vi "Teleop.vi"(8 "Ramps":bool, 9 "Shift":bool, 10 "Match Info":T1={"Autonomous Elapsed Seconds"=0.0, "TeleOp Elapsed Seconds"=0.0, "Disabled Elapsed Seconds"=0.0, "Visited Autonomous"=FALSE, "Visited TeleOp"=FALSE, "Visited Disabled"=FALSE, "Autonomous Settings"={"Autonomous Style"=enum."Independent", "VI Refnum"=refnum}}, 11 "Call Context":T2) -> ()   [LabVIEW 2017]
doc: "This VI is called for each TeleOp packet received from the DS where the robot is not disabled. It is often used to read from the joysticks and update I/O or to update setpoints for timed control loops. It should complete and return within 20 milliseconds or it may miss DS packets."
uses:
  <vilib>/Rock Robotics/WPI/DriverStation/WPI_DriverStationDerivedRobotMode.ctl
  <vilib>/Rock Robotics/WPI/DriverStation/WPI_DriverStationMatch Info.ctl
  <vilib>/Rock Robotics/WPI/Solenoid/WPI_SolenoidValue.ctl
  Public/Documents/Cross The Road Electronics/Phoenix-LabVIEW/Motor Controller/Controls/CTRE_Phoenix_MotorControl_ControlMode.ctl
  <vilib>/Rock Robotics/WPI/Utilities/WPI_GetSetVariantRefNum.vi
  <vilib>/Rock Robotics/Network Tables/NT Write Boolean Array.vi
  <vilib>/Rock Robotics/Network Tables/NT Write Numeric Array.vi
  <vilib>/Rock Robotics/Network Tables/NT Read Boolean.vi
  <vilib>/Rock Robotics/Network Tables/NT Read Numeric Array.vi
  <vilib>/Rock Robotics/Network Tables/NT Read Boolean Array.vi
  <vilib>/Rock Robotics/Network Tables/NT Write Number.vi
  <vilib>/Rock Robotics/WPI/Joystick/WPI_JoystickArcadeMapping.vi
  <vilib>/Rock Robotics/WPI/RobotDrive/WPI_RobotDriveArcadeDrive_Standard(NoSaturation).vi
  <vilib>/Rock Robotics/WPI/ThirdParty/Phoenix-LabVIEW/Motor Controller/Controls/CTRE_Phoenix_MotorControl_NeutralMode.ctl
panel:
  out "element":dbl
  in  "L Retract Ramps":bool
  in  "R Retract Ramps":bool
  in  "RRamp Raise":bool
  in  "LRamp Raise":bool=TRUE
  in  "RRamp Deploy":bool
  in  "LRamp Deploy":bool
  in  "Cube Down":bool
  in  "Cube Up":bool
  in  "Direction Toggle":bool
  in  "Gear Shift":bool
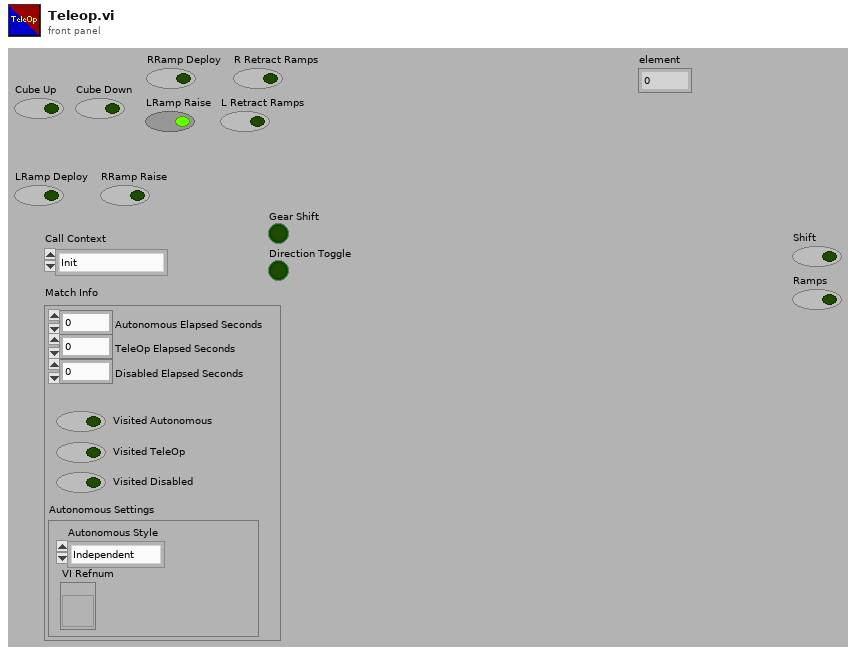
[diagram p1: front panel]
types:
  T1 = typedef "WPI_DriverStationMatch Info.ctl" = cluster{"Autonomous Elapsed Seconds":dbl, "TeleOp Elapsed Seconds":dbl, "Disabled Elapsed Seconds":dbl, "Visited Autonomous":bool, "Visited TeleOp":bool, "Visited Disabled":bool, "Autonomous Settings":cluster{"Autonomous Style":enum16{"Iterative", "Independent"}, "VI Refnum":refnum<vi>}}
  T2 = typedef "WPI_DriverStationDerivedRobotMode.ctl" = enum16{"Init", "Execute", "Stop"}
  T3 = typedef "CTRE_Phoenix_MotorControl_ControlMode.ctl" = u16
  T4 = typedef "WPI_SolenoidValue.ctl" = enum16{"Off", "On", "Forward", "Reverse"}
  T5 = typedef "WPI_JoystickDevRef.ctl" = cluster{"Device":T6}
  T6 = typedef "WPI_JoystickDeviceEnum.ctl" = enum16{"USB 0", "USB 1", "USB 2", "USB 3", "USB 4", "USB 5"}
  T7 = typedef "CTRE_Phoenix_MotorControl_NeutralMode.ctl" = enum8{"EEPROMSetting", "Override to Coast", "Override to Brake"}
  T8 = typedef "WPI_MotorControlDeviceRef.ctl" = cluster{"DeviceStatus":errorcluster, "Type":T9, "PWM":cluster{"PWM Channel":T10, "DeadBand":T11}, "CAN":cluster{"Device Number":u8, "SetOutput VI Ref":variant, "GetOutput VI Ref":variant, "Enable VI Ref":variant, "Disable VI Ref":variant, "Data":variant}, "Invert":bool, "DIO PWM":cluster{"PWM \"Enable\" Channel":T10, "DIOChannel":T12, "PWM Rate":dbl}}
  T9 = typedef "WPI_MotorControlType.ctl" = enum16{"PWM", "CAN", "DIO PWM"}
  T10 = typedef "FPGA_DIOPWMChannel.ctl" = enum8{"PWM 0", "PWM 1", "PWM 2", "PWM 3", "PWM 4", "PWM 5", "PWM 6", "PWM 7", "PWM 8", "PWM 9", "PWM MXP 0", "PWM MXP 1", "PWM MXP 2", "PWM MXP 3", "PWM MXP 4", "PWM MXP 5", "PWM MXP 6", "PWM MXP 7", "PWM MXP 8", "PWM MXP 9", "Invalid"}
  T11 = typedef "WPI_PWMDeadband.ctl" = cluster{"Name":string, "maxPositivePwm":i32, "minPositivePwm":i32, "centerPwm":i32, "maxNegativePwm":i32, "minNegativePwm":i32, "angularRange":u16}
  T12 = typedef "FPGA_DIOChannel.ctl" = enum8{"DIO 0", "DIO 1", "DIO 2", "DIO 3", "DIO 4", "DIO 5", "DIO 6", "DIO 7", "DIO 8", "DIO 9", "DIO MXP 0", "DIO MXP 1", "DIO MXP 2", "DIO MXP 3", "DIO MXP 4", "DIO MXP 5", "DIO MXP 6", "DIO MXP 7", "DIO MXP 8", "DIO MXP 9", "DIO MXP 10", "DIO MXP 11", "DIO MXP 12", "DIO MXP 13", "DIO MXP 14", "DIO MXP 15", "SPI Port CS1", "SPI Port CS2", "SPI Port CS3", "SPI Port MISO", "SPI Port MOSI", "Invalid"}
  T13 = typedef "WPI_RobotDriveDevRef.ctl" = cluster{"DevStatus":errorcluster, "Motors[]":T8[], "Square Inputs":bool, "Max Output":dbl}
  T14 = typedef "WPI_SolenoidDevRef.ctl" = cluster{"DevStatus":errorcluster, "Pneumatics Control Module":u8, "Forward Solenoid Channel":T15, "Reverse Solenoid Channel":T15}
  T15 = typedef "WPI_SolenoidChannel.ctl" = enum8{"Solenoid 0", "Solenoid 1", "Solenoid 2", "Solenoid 3", "Solenoid 4", "Solenoid 5", "Solenoid 6", "Solenoid 7", "Invalid"}
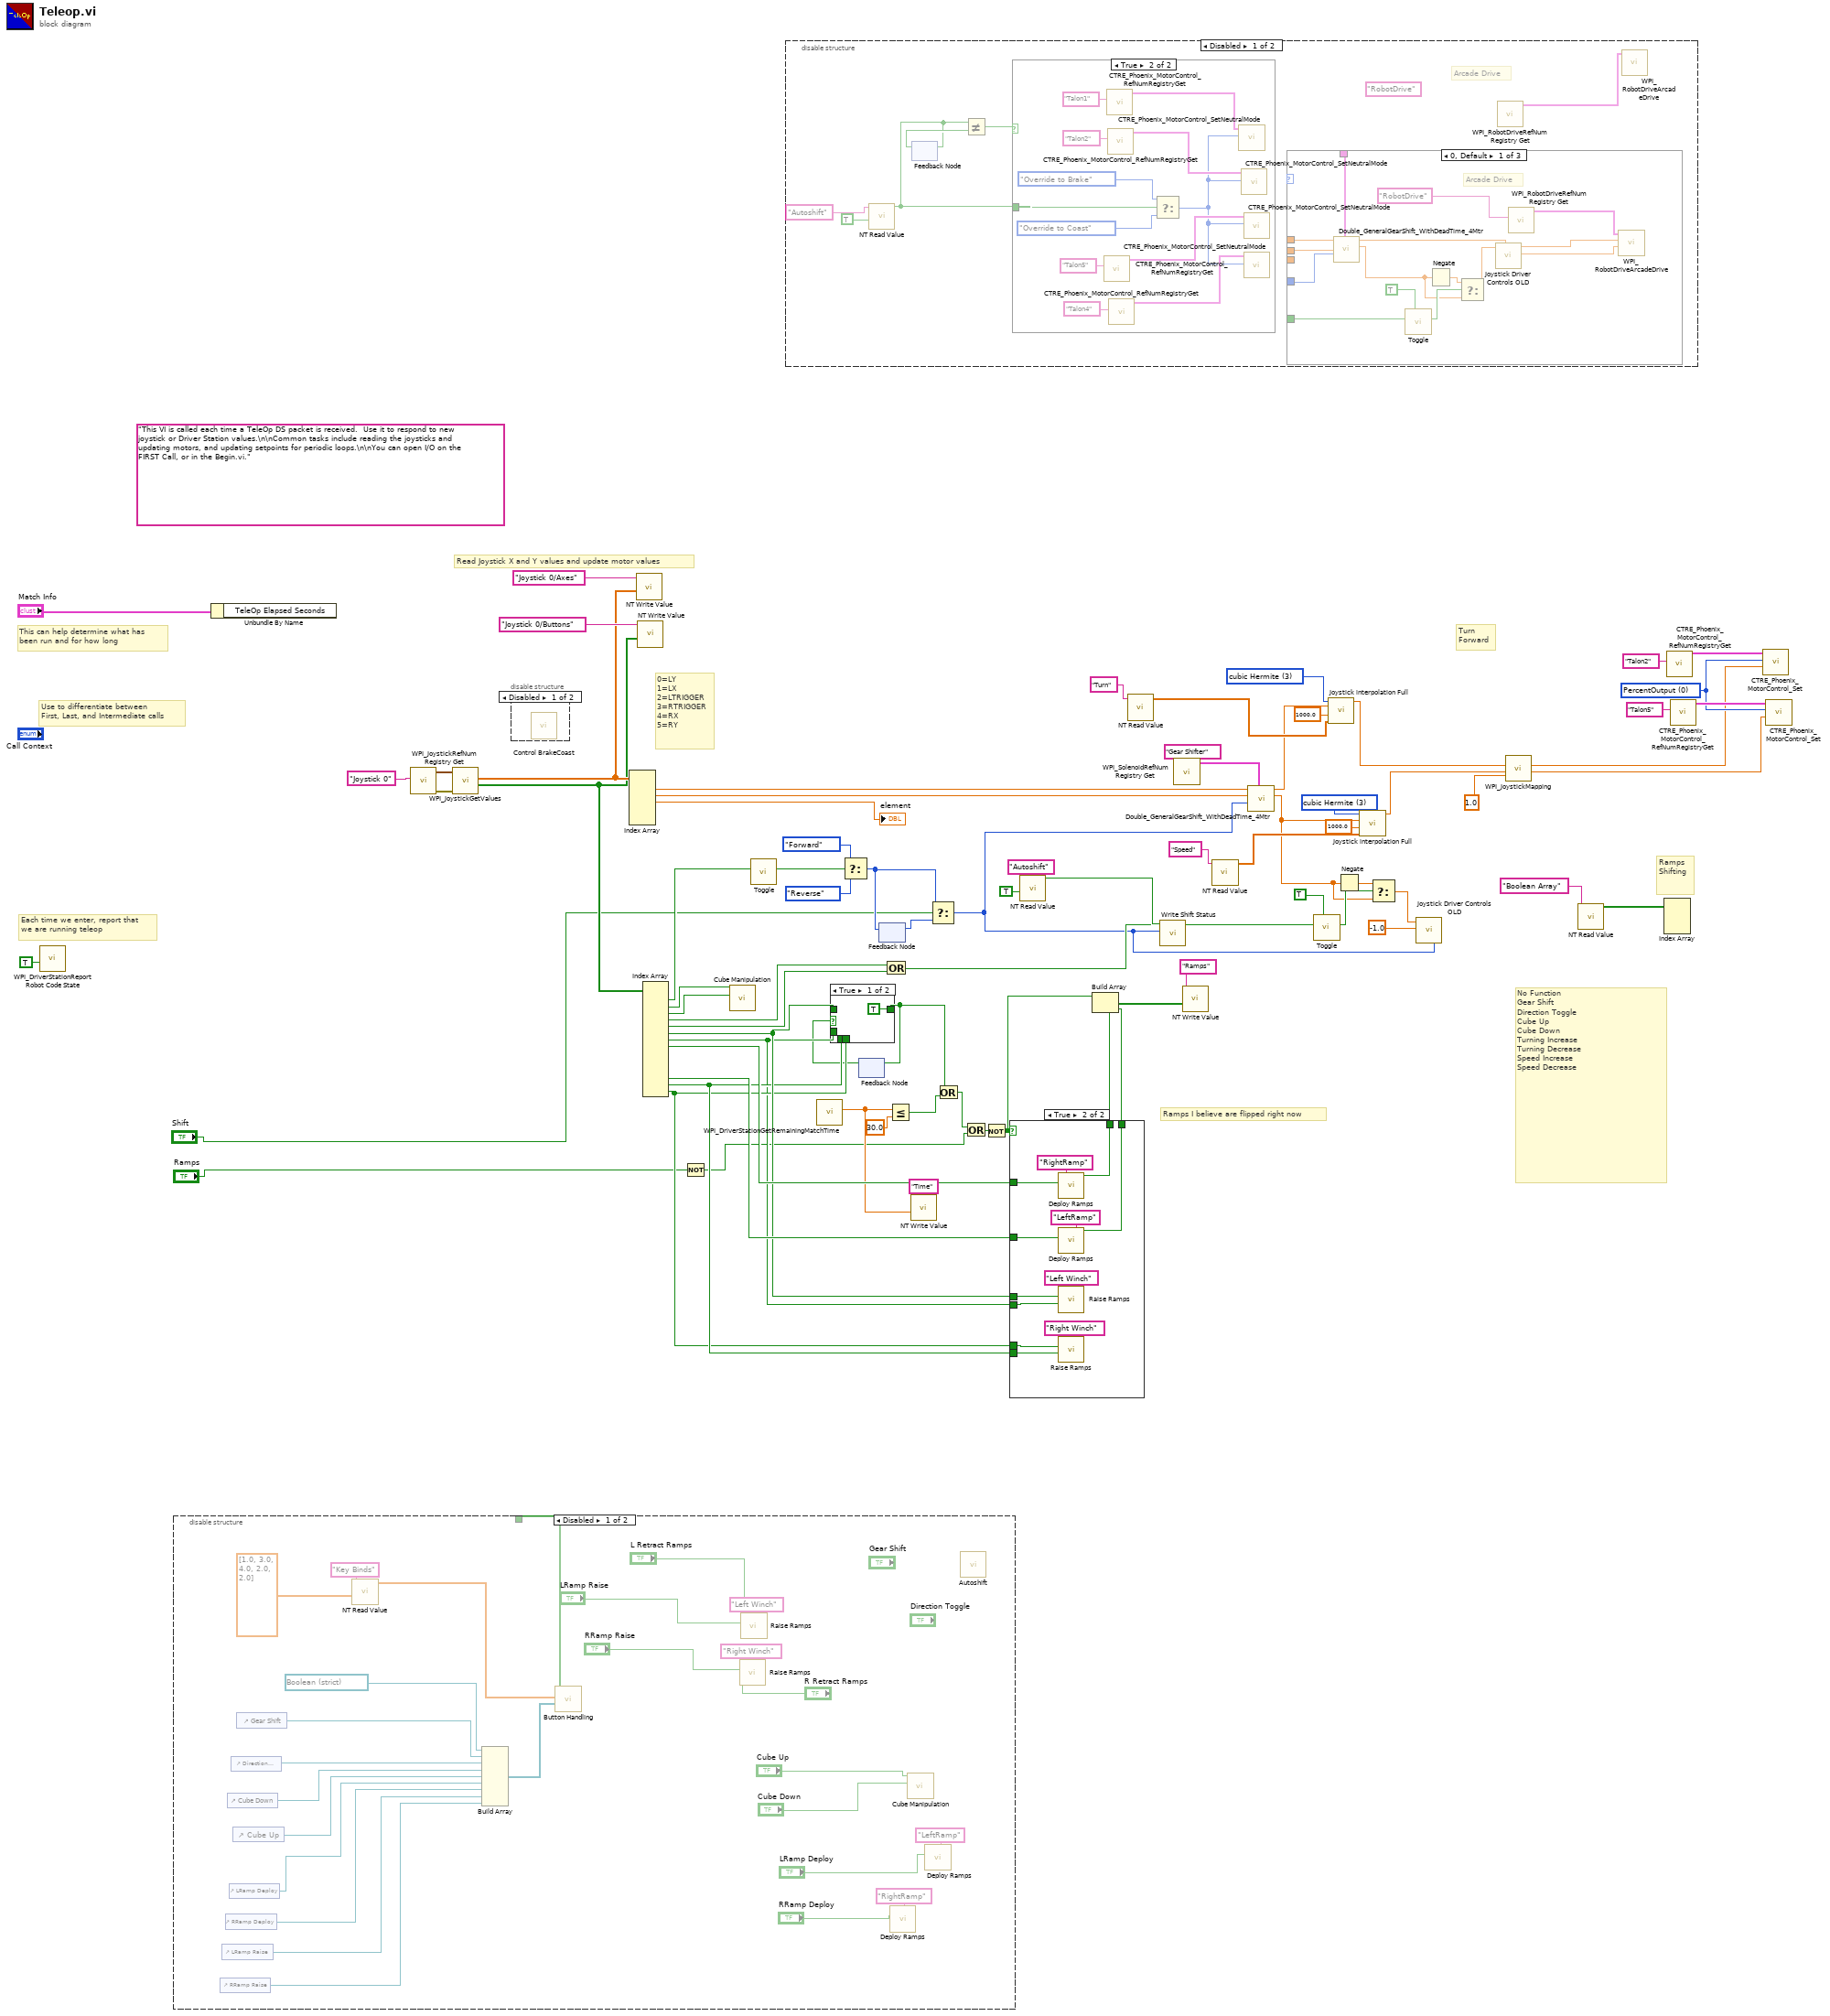
[diagram p0: block diagram]
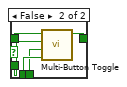
[diagram p2: hidden frame]
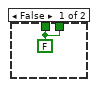
[diagram p3: hidden frame]
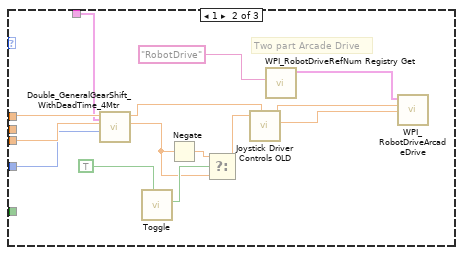
[diagram p5: hidden frame]
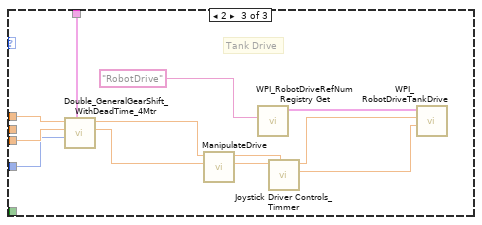
[diagram p6: hidden frame]
diagram:
  w12 = 3 items=["nearest", "linear", "spline", "cubic Hermite", "Lagrange"] ("method")
  w19 = 3 items=["nearest", "linear", "spline", "cubic Hermite", "Lagrange"] ("method")
  w42 = T3 0 items=["PercentOutput"=0, "Position"=1, "Velocity"=2, "Current"=3, "Follower"=5, "MotionProfile"=6, "MotionMagic"=7, "MotionMagicArc"=8, "MotionProfileArc"=10, "Disabled"=15] ("Control Mode")
  (unwired) "This VI is called each time a TeleOp DS packet is received.  Use it to respond to new joystick or Driver Station values.\n\nCommon tasks include reading the joysticks and updating motors, and updating setpoints for periodic loops.\n\nYou can open I/O on the FIRST Call, or in the Begin.vi."
  # "Ramps\nShifting"
  # "Turn\nForward"
  # "Ramps I believe are flipped right now"
  # "No Function\nGear Shift\nDirection Toggle\nCube Up\nCube Down\nTurning Increase\nTurning Decrease\nSpeed Increase\nSpeed Decrease"
  # "0=LY\n1=LX\n2=LTRIGGER\n3=RTRIGGER\n4=RX\n5=RY"
  # "Each time we enter, report that\nwe are running teleop"
  # "Use to differentiate between\nFirst, Last, and Intermediate calls"
  # "This can help determine what has\nbeen run and for how long"
  # "Read Joystick X and Y values and update motor values"
  n1 = call <vilib>:"WPI_DriverStationReport Robot Code State.vi"("TeleOp"=TRUE ("Autonomous")) -> ()  [unwired: 10 in, 1 out]
  n2 = disable-structure shown="Disabled" {
    disable-tunnel: _ -> [w81 _]
    frame Disabled {
      n3 = control-ref of="RRamp Raise"() -> (w95:refnum<vi>)
      n4 = control-ref of="LRamp Raise"() -> (w96:refnum<vi>)
      n5 = control-ref of="RRamp Deploy"() -> (w98:refnum<vi>)
      n6 = control-ref of="Cube Down"() -> (w101:refnum<vi>)
      n7 = control-ref of="LRamp Deploy"() -> (w99:refnum<vi>)
      n8 = control-ref of="Direction Toggle"() -> (w103:refnum<vi>)
      n9 = control-ref of="Cube Up"() -> (w100:refnum<vi>)
      n10 = control-ref of="Gear Shift"() -> (w104:refnum<vi>)
      n11 = call-poly <vilib>:"NT Read Value.vi"("Default Value"=dbl[] [1.0, 3.0, 4.0, 2.0, 2.0], "Name"="Key Binds") -> ("Numeric Array"=w80:dbl[])  [unwired: 8 in, 1 out]
      n12 = Build Array(refnum<vi> refnum ("element"), w104, w103, w101, w100, w99, w98, w96, w95) -> (w79:refnum<vi>[])
      n13 = call "Button Handling.vi"("Array"=w79, "Numeric Array"=w80, "Buttons"=w81) -> ()  [unwired: 9 in]
      n14 = call "Raise Ramps.vi"("Retract Ramps"="R Retract Ramps", "Raise Ramps"="RRamp Raise", "refnum name"="Right Winch") -> ()  [unwired: 9 in]
      n15 = call "Raise Ramps.vi"("Retract Ramps"="L Retract Ramps", "Raise Ramps"="LRamp Raise", "refnum name"="Left Winch") -> ()  [unwired: 9 in]
      n16 = call "Deploy Ramps.vi"("Deploy"="RRamp Deploy", "refnum name"="RightRamp") -> ()  [unwired: 9 in, 1 out]
      n17 = call "Cube Manipulation.vi"("Outtake"="Cube Down", "Intake"="Cube Up") -> ()  [unwired: 10 in]
      n18 = call "Deploy Ramps.vi"("Deploy"="LRamp Deploy", "refnum name"="LeftRamp") -> ()  [unwired: 9 in, 1 out]
      n19 = call "Autoshift.vi"() -> ()  [unwired: 12 in]
    }
    frame Enabled {
    }
  }
  n20 = Unbundle By Name("Match Info") -> ()  [unwired: 1 out]
  n21 = call <vilib>:"WPI_JoystickRefNum Registry Get.vi"("refnum name"="Joystick 0") -> ("error out"=w63:errorcluster, "JoystickDevRef"=w77:T5)  [unwired: 1 in, 8 out]
  n22 = call <vilib>:"WPI_JoystickGetValues.vi"("error in (no error)"=w63, "JoystickDevRef"=w77) -> ("Buttons"=w62:bool[], "Axes"=w73:dbl[])  [unwired: 5 in, 3 out]
  n23 = disable-structure shown="Disabled" {
    frame Disabled {
      n24 = call "Control BrakeCoast.vi"() -> ()  [unwired: 12 in]
    }
    frame Enabled {
    }
  }
  n25 = Index Array(array=w73) -> (element #1=w72:dbl, element #2=w71:dbl, element #3=→"element":dbl)  [unwired: 6 in, 3 out]
  n26 = call-poly <vilib>:"NT Write Value.vi"("Numeric Array"=w73, "Name"="Joystick 0/Axes") -> ()  [unwired: 9 in, 1 out]
  n27 = call-poly <vilib>:"NT Write Value.vi"("Boolean Array"=w62, "Name"="Joystick 0/Buttons") -> ()  [unwired: 9 in, 1 out]
  n28 = Index Array(array=w62) -> (element #1=w53:bool, element #2=w54:bool, element #3=w55:bool, element #4=w48:bool, element #5=w49:bool, element #6=w34:bool, element #7=w31:bool, element #8=w40:bool, element #9=w41:bool, element #10=w33:bool, element #11=w32:bool)  [unwired: 15 in, 4 out]
  n29 = Not(x="Ramps") -> (.not. x?=w9:bool)
  n30 = call "Cube Manipulation.vi"("Outtake"=w55, "Intake"=w54) -> ()  [unwired: 10 in]
  n31 = call "Toggle.vi"("Input"=w53) -> ("Output"=w69:bool)  [unwired: 10 in]
  n32 = disable-structure shown="Disabled" {
    frame Disabled {
      (unwired) "RobotDrive" ("refnum name")
      # "Arcade Drive"
      n33 = call-poly <vilib>:"NT Read Value.vi"("Default Value"=TRUE, "Name"="Autoshift") -> ("Boolean"=w107:bool)  [unwired: 8 in, 1 out]
      n34 = feedback #1() -> (w108:bool)  [unwired: 1 in]
      n35 = feedback-in #1(w107) -> ()
      n36 = Not Equal?(x=w107, y=w108) -> (x != y?=w106:bool)
      n37 = case shown="True" w106 {
        tunnel: w107 -> [_ w159]
        frame False {
        }
        frame True {
          n38 = call <vilib>:"CTRE_Phoenix_MotorControl_RefNumRegistryGet.vi"("refnum name"="Talon5") -> ("PhoenixMotorControlDevRef"=w160:T8)  [unwired: 9 in, 1 out]
          n39 = call <vilib>:"CTRE_Phoenix_MotorControl_RefNumRegistryGet.vi"("refnum name"="Talon1") -> ("PhoenixMotorControlDevRef"=w152:T8)  [unwired: 9 in, 1 out]
          n40 = call <vilib>:"CTRE_Phoenix_MotorControl_RefNumRegistryGet.vi"("refnum name"="Talon2") -> ("PhoenixMotorControlDevRef"=w161:T8)  [unwired: 9 in, 1 out]
          n41 = call <vilib>:"CTRE_Phoenix_MotorControl_RefNumRegistryGet.vi"("refnum name"="Talon4") -> ("PhoenixMotorControlDevRef"=w154:T8)  [unwired: 9 in, 1 out]
          n42 = Select(t=CTRE_Phoenix_MotorControl_NeutralMode."Override to Brake" ("Motor Control Neutral Mode"), s=w159, f=CTRE_Phoenix_MotorControl_NeutralMode."Override to Coast" ("Motor Control Neutral Mode")) -> (s? t:f=w153:T7)
          n43 = call <vilib>:"CTRE_Phoenix_MotorControl_SetNeutralMode.vi"("Motor Control Neutral Mode"=w153, "PhoenixMotorControlDevRef"=w152) -> ()  [unwired: 8 in, 2 out]
          n44 = call <vilib>:"CTRE_Phoenix_MotorControl_SetNeutralMode.vi"("Motor Control Neutral Mode"=w153, "PhoenixMotorControlDevRef"=w161) -> ()  [unwired: 8 in, 2 out]
          n45 = call <vilib>:"CTRE_Phoenix_MotorControl_SetNeutralMode.vi"("Motor Control Neutral Mode"=w153, "PhoenixMotorControlDevRef"=w160) -> ()  [unwired: 8 in, 2 out]
          n46 = call <vilib>:"CTRE_Phoenix_MotorControl_SetNeutralMode.vi"("Motor Control Neutral Mode"=w153, "PhoenixMotorControlDevRef"=w154) -> ()  [unwired: 8 in, 2 out]
        }
      }
      n47 = case shown="0, Default" {
        selector: _ -> [_ _ _]
        tunnel: _ -> [w119 w131 w144]
        tunnel: _ -> [_ w130 w143]
        tunnel: _ -> [w118 _ _]
        tunnel: _ -> [w115 w126 w142]
        tunnel: _ -> [w114 w127 w145]
        tunnel: _ -> [w111 _ _]
        frame 0, Default {
          # "Arcade Drive"
          n48 = call "Double_GeneralGearShift_WithDeadTime_4Mtr.vi"("ShifterRef"=w114, "Shift Value"=w115, "Right"=w118, "Left"=w119) -> ("Right Output"=w116:dbl, "Left Output"=w117:dbl)  [unwired: 4 in, 2 out]
          n49 = call "Toggle.vi"("Control"=TRUE, "Input"=w111) -> ("Output"=w123:bool)  [unwired: 9 in]
          n50 = Negate(x=w116) -> (-x=w122:dbl)
          n51 = Select(t=w122, s=w123, f=w116) -> (s? t:f=w120:dbl)
          n52 = call "Joystick Driver Controls OLD.vi"("X"=w117, "Y"=w120) -> ("Y"=w113:dbl, "X"=w112:dbl)  [unwired: 8 in]
          n53 = call <vilib>:"WPI_RobotDriveRefNum Registry Get.vi"("refnum name"="RobotDrive") -> ("RobotDriveDevRef"=w124:T13)  [unwired: 9 in, 1 out]
          n54 = call-poly <vilib>:"WPI_RobotDriveArcadeDrive.vi"("Y axis value"=w113, "X axis value"=w112, "RobotDriveDevRef"=w124) -> ()  [unwired: 6 in, 3 out]
        }
        frame 1 {
          # "Two part Arcade Drive"
          n55 = call "Double_GeneralGearShift_WithDeadTime_4Mtr.vi"("ShifterRef"=w127, "Shift Value"=w126, "Right"=w130, "Left"=w131) -> ("Right Output"=w128:dbl, "Left Output"=w129:dbl)  [unwired: 4 in, 2 out]
          n56 = call "Toggle.vi"("Control"=TRUE) -> ("Output"=w135:bool)  [unwired: 10 in]
          n57 = Negate(x=w128) -> (-x=w134:dbl)
          n58 = Select(t=w134, s=w135, f=w128) -> (s? t:f=w132:dbl)
          n59 = call "Joystick Driver Controls OLD.vi"("X"=w129, "Y"=w132) -> ("Y"=w136:dbl, "X"=w137:dbl)  [unwired: 8 in]
          n60 = call <vilib>:"WPI_RobotDriveRefNum Registry Get.vi"("refnum name"="RobotDrive") -> ("RobotDriveDevRef"=w138:T13)  [unwired: 9 in, 1 out]
          n61 = call-poly <vilib>:"WPI_RobotDriveArcadeDrive.vi"("Y axis value"=w136, "X axis value"=w137, "RobotDriveDevRef"=w138) -> ()  [unwired: 6 in, 3 out]
        }
        frame 2 {
          # "Tank Drive"
          n62 = call "Double_GeneralGearShift_WithDeadTime_4Mtr.vi"("ShifterRef"=w145, "Shift Value"=w142, "Right"=w143, "Left"=w144) -> ("Right Output"=w141:dbl, "Left Output"=w140:dbl)  [unwired: 4 in, 2 out]
          n63 = call "ManipulateDrive.vi"("Y"=w141, "X"=w140) -> ("Y"=w148:dbl, "X"=w149:dbl)  [unwired: 4 in]
          n64 = call <vilib>:"WPI_RobotDriveRefNum Registry Get.vi"("refnum name"="RobotDrive") -> ("RobotDriveDevRef"=w150:T13)  [unwired: 9 in, 1 out]
          n65 = call "Joystick Driver Controls_Timmer.vi"("X"=w149, "Y"=w148) -> ("Y"=w146:dbl, "X"=w147:dbl)  [unwired: 8 in]
          n66 = call <vilib>:"WPI_RobotDriveTankDrive.vi"("Right axis value"=w146, "Left axis value"=w147, "RobotDriveDevRef"=w150) -> ()  [unwired: 6 in, 3 out]
        }
      }
      n67 = call <vilib>:"WPI_RobotDriveRefNum Registry Get.vi"() -> ("RobotDriveDevRef"=w105:T13)  [unwired: 10 in, 1 out]
      n68 = call-poly <vilib>:"WPI_RobotDriveArcadeDrive.vi"("RobotDriveDevRef"=w105) -> ()  [unwired: 8 in, 3 out]
    }
    frame Enabled {
    }
  }
  n69 = call <vilib>:"WPI_DriverStationGetRemainingMatchTime.vi"() -> ("Match Time(s)"=w30:sgl)  [unwired: 10 in, 1 out]
  n70 = Select(t=WPI_SolenoidValue."Forward" ("Shift Value"), s=w69, f=WPI_SolenoidValue."Reverse" ("Shift Value")) -> (s? t:f=w5:T4)
  n71 = feedback #2() -> (w26:bool)  [unwired: 1 in]
  n72 = case shown="True" w26 {
    tunnel: w34 -> [_ w169]
    tunnel: w33 -> [_ w168]
    tunnel: w32 -> [_ w167]
    tunnel: w31 -> [_ w166]
    tunnel: [TRUE ("Output") w165] -> w27
    frame True {
    }
    frame False {
      n73 = call "Multi-Button Toggle.vi"("Button 4"=w168, "Button 3"=w167, "Button 2"=w166, "Button 1"=w169) -> ("Output"=w165:bool)  [unwired: 7 in]
    }
  }
  n74 = feedback-in #2(w27) -> ()
  n75 = feedback-in #3(w5) -> ()
  n76 = feedback #3() -> (w7:T4)  [unwired: 1 in]
  n77 = Or(x=w48, y=w49) -> (x .or. y?=w50:bool)
  n78 = Less Or Equal?(x=w30, y=sgl 30.0) -> (x <= y?=w28:bool)
  n79 = call-poly <vilib>:"NT Write Value.vi"("Numeric"=w30, "Name"="Time") -> ()  [unwired: 9 in, 1 out]
  n80 = Select(t=w5, s="Shift", f=w7) -> (s? t:f=w6:T4)
  n81 = Or(x=w27, y=w28) -> (x .or. y?=w1:bool)
  n82 = Or(x=w1, y=w9) -> (x .or. y?=w8:bool)
  n83 = Not(x=w8) -> (.not. x?=w2:bool)
  n84 = case shown="True" w2 {
    tunnel: w34 -> [_ w178]
    tunnel: w31 -> [_ w177]
    tunnel: w40 -> [_ w176]
    tunnel: w41 -> [_ w175]
    tunnel: w33 -> [_ w174]
    tunnel: w32 -> [_ w173]
    tunnel: [w170 w172] -> w37
    tunnel: [w170 w171] -> w36
    frame False {
      w170 = FALSE ("Output")
    }
    frame True {
      n85 = call "Deploy Ramps.vi"("Deploy"=w176, "refnum name"="RightRamp") -> ("Output"=w172:bool)  [unwired: 9 in]
      n86 = call "Deploy Ramps.vi"("Deploy"=w175, "refnum name"="LeftRamp") -> ("Output"=w171:bool)  [unwired: 9 in]
      n87 = call "Raise Ramps.vi"("Retract Ramps"=w177, "Raise Ramps"=w178, "refnum name"="Left Winch") -> ()  [unwired: 9 in]
      n88 = call "Raise Ramps.vi"("Retract Ramps"=w174, "Raise Ramps"=w173, "refnum name"="Right Winch") -> ()  [unwired: 9 in]
    }
  }
  n89 = call-poly <vilib>:"NT Read Value.vi"("Default Value"=TRUE, "Name"="Autoshift") -> ("Boolean"=w51:bool)  [unwired: 8 in, 1 out]
  n90 = Build Array(w2, w37, w36) -> (w39:bool[])
  n91 = call-poly <vilib>:"NT Read Value.vi"("Name"="Turn") -> ("Numeric Array"=w13:dbl[])  [unwired: 9 in, 1 out]
  n92 = call "Write Shift Status.vi"("Gear"=w6, "Autoshifting"=w51) -> ()  [unwired: 9 in, 1 out]
  n93 = call <vilib>:"WPI_SolenoidRefNum Registry Get.vi"("refnum name"="Gear Shifter") -> ("SolenoidDevRef"=w66:T14)  [unwired: 9 in, 1 out]
  n94 = call-poly <vilib>:"NT Write Value.vi"("Boolean Array"=w39, "Name"="Ramps") -> ()  [unwired: 9 in, 1 out]
  n95 = call-poly <vilib>:"NT Read Value.vi"("Name"="Speed") -> ("Numeric Array"=w20:dbl[])  [unwired: 9 in, 1 out]
  n96 = call "Double_GeneralGearShift_WithDeadTime_4Mtr.vi"("ShifterRef"=w66, "Shift Value"=w6, "Right"=w71, "Left"=w72) -> ("Right Output"=w16:dbl, "Left Output"=w11:dbl)  [unwired: 4 in, 2 out]
  n97 = call "Toggle.vi"("Control"=TRUE, "Input"=w50) -> ("Output"=w61:bool)  [unwired: 9 in]
  n98 = call "Joystick interpolation Full.vi"("array"=w13, "Numeric"=1000.0, "Joystick Sim"=w11, "method"=w12) -> ("Power"=w10:dbl)  [unwired: 7 in]
  n99 = Negate(x=w16) -> (-x=w60:dbl)
  n100 = call "Joystick interpolation Full.vi"("array"=w20, "Numeric"=1000.0, "Joystick Sim"=w16, "method"=w19) -> ("Power"=w17:dbl)  [unwired: 7 in]
  n101 = Select(t=w60, s=w61, f=w16) -> (s? t:f=w58:dbl)
  n102 = call "Joystick Driver Controls OLD.vi"("Shift Value"=w6, "Throttle"=-1.0, "Y"=w58) -> ()  [unwired: 7 in, 2 out]
  n103 = call-poly <vilib>:"WPI_JoystickMapping.vi"("Max Output"=1.0, "Y axis value"=w17, "X axis value"=w10) -> ("Right Motor Value"=w24:dbl, "Left Motor Value"=w25:dbl)  [unwired: 7 in]
  n104 = call-poly <vilib>:"NT Read Value.vi"("Name"="Boolean Array") -> ("Boolean Array"=w22:bool[])  [unwired: 9 in, 1 out]
  n105 = Index Array(array=w22) -> ()  [unwired: 3 in, 3 out]
  n106 = call <vilib>:"CTRE_Phoenix_MotorControl_RefNumRegistryGet.vi"("refnum name"="Talon2") -> ("PhoenixMotorControlDevRef"=w44:T8)  [unwired: 9 in, 1 out]
  n107 = call <vilib>:"CTRE_Phoenix_MotorControl_RefNumRegistryGet.vi"("refnum name"="Talon5") -> ("PhoenixMotorControlDevRef"=w43:T8)  [unwired: 9 in, 1 out]
  n108 = call <vilib>:"CTRE_Phoenix_MotorControl_Set.vi"("Output"=w25, "Control Mode"=w42, "PhoenixMotorControlDevRef"=w44) -> ()  [unwired: 7 in, 2 out]
  n109 = call <vilib>:"CTRE_Phoenix_MotorControl_Set.vi"("Output"=w24, "Control Mode"=w42, "PhoenixMotorControlDevRef"=w43) -> ()  [unwired: 7 in, 2 out]
